vi "WPI_CounterWARNDigitalSourceAndEdgeType.vi"() -> (0 "WARNDigitalSourceAndEdgeType":errorcluster)   [LabVIEW 2017]
doc: "This software is licensed. Open the labview\\readme\\WPI Robotics Library Open Source License.txt file for more information."
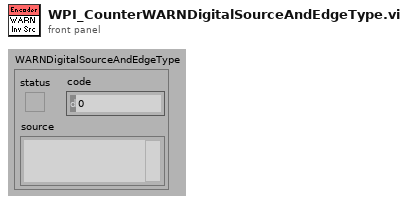
[diagram p1: front panel]
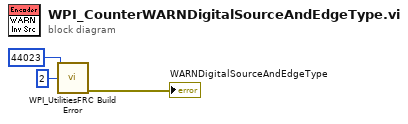
[diagram p0: block diagram]
diagram:
  n1 = call <vilib>:"WPI_UtilitiesFRC Build Error.vi"("error code"=44023 ("code"), "chain levels to remove (1)"=2) -> ("error out"=→"WARNDigitalSourceAndEdgeType":errorcluster)  [unwired: 3 in, 10 out]
